vi "register upgrade handler.vi"(8 "error in":errorcluster, 9 "callback":T1, 10 "protocol":string, 11 "http responder in":refnum<class "https responder.lvclass">) -> (0 "error out":errorcluster, 3 "http responder out":refnum<class "https responder.lvclass">)   [LabVIEW 2016, in "https responder.lvclass"]
uses:
  https responder.lvclass
  http upgrade callback.ctl
  lvlibtls/socket connection/lvlibretls connection.lvclass
  https responder.lvclass/https responder.ctl
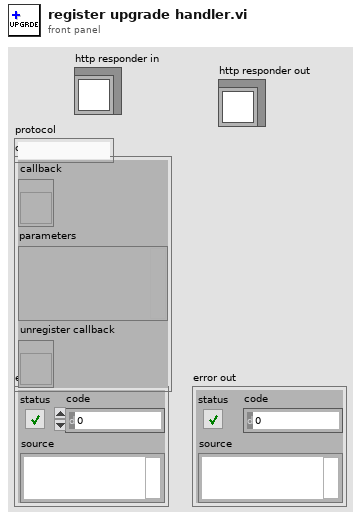
[diagram p1: front panel]
types:
  T1 = typedef "https responder.lvclass/http upgrade callback.ctl" = cluster{"callback":refnum<vi>, "parameters":variant, "unregister callback":refnum<vi>}
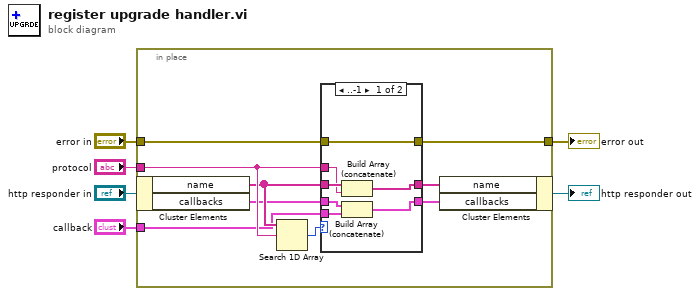
[diagram p0: block diagram]
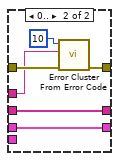
[diagram p2: hidden frame]
diagram:
  n1 = in-place {
    in-place-border: "protocol" -> [w12]
    in-place-border: "error in" -> [w14]
    in-place-border: [w13] -> w2
    in-place-border: "callback" -> [w7]
    n2 = in-place-cluster #1("http responder in") -> ("name"=w11:string[], "callbacks"=w9:T1[])
    n3 = Search 1D Array(1D array=w11, element=w12) -> (index of element=w15:i32)  [unwired: 1 in]
    n4 = case shown="..-1" w15 {
      tunnel: w14 -> [w19 w28]
      tunnel: [w19 w27] -> w13
      tunnel: w12 -> [w16 w25]
      tunnel: w11 -> [w17 w24]
      tunnel: [w18 w24] -> w10
      tunnel: w9 -> [w22 w23]
      tunnel: [w20 w23] -> w8
      tunnel: w7 -> [w21 _]
      frame ..-1 {
        n5 = Build Array (concatenate)(w17, w16) -> (w18:string[])
        n6 = Build Array (concatenate)(w22, w21) -> (w20:T1[])
      }
      frame 0.. {
        n7 = call <vilib>:"Error Cluster From Error Code.vi"("error in (no error)"=w28, "error message (\"\")"=w25, "error code (0)"=10) -> ("error out"=w27:errorcluster)  [unwired: 6 in]
      }
    }
    n8 = in-place-cluster #1("name"=w10, "callbacks"=w8) -> (→"http responder out":refnum<class "https responder.lvclass">)
  }
  "error out" <- w2
